vi "RT Driver VI.vi"(7 "Operation":T1, 11 "Device Reference in":T2 format="%.0x") -> (0 "Error Code":i32)   [LabVIEW 2016, in "FPGA Addon Engine.lvlib"]
uses:
  FPGA Addon Engine.lvlib
  <vilib>/NI Veristand/Custom Device API/Custom Device Item Ref.ctl
  <vilib>/NI Veristand/Custom Device API/Hardware Interface Driver VI Operation.ctl
  <vilib>/NI/NIVS Inline Async API/_VS Inline Async API/VS Inline Async API/VS Inline Async API.lvclass/VS Inline Async API.ctl
  <vilib>/NI/NIVS Inline Async API/_Data Access Engine/Data Access Engine/Data Access Engine.lvclass/Data Access Engine.ctl
  <vilib>/NI/NIVS Inline Async API/_Data Access Engine/Access Type Classes/Write/Write.lvclass/Write.ctl
  <vilib>/NI/NIVS Inline Async API/_Data Access Engine/Access Type Classes/ReadWrite/ReadWrite.lvclass/ReadWrite.ctl
  FPGA-Resource-Manager-APIs/Source/Shared/FPGA Settings.vi
  SubVIs/Initialize Scalar Datatypes and Refs.vi
  <vilib>/NI/NIVS Inline Async API/_Data Access Engine/Data Access Engine/Methods/Data.Engine.Read Data from HW.vi
  <vilib>/NI/NIVS Inline Async API/_VS Inline Async API/Error Handling Process/SubVIs/Error.GetError.vi
  <vilib>/NI/NIVS Inline Async API/_Data Access Engine/Access Type Classes/ReadWrite/ReadWrite.EngineData.vi
  <vilib>/NI/NIVS Inline Async API/_Data Access Engine/Access Type Classes/Write/Write.EngineData.vi
  <vilib>/NI Veristand/Custom Device API/NI VeriStand - Get Channel Value by Data Reference.vi
  <vilib>/NI Veristand/Custom Device API/NI VeriStand - Set Channel Value by Data Reference.vi
  <vilib>/Utility/config.llb/Open Config Data.vi
  <vilib>/Utility/config.llb/Get Key Names.vi
  <vilib>/Utility/config.llb/Write Key.vi
  <vilib>/Utility/config.llb/Write Key (I32).vi
  <vilib>/Utility/config.llb/Close Config Data.vi
  Shared/Constants.vi
  <vilib>/NI Veristand/Custom Device API/NI VeriStand - Get Item Property.vi
  <vilib>/NI Veristand/Custom Device API/Get Item Property (Variant).vi
  <vilib>/NI Veristand/Custom Device API/Get Item Property (Dependent File).vi
  <vilib>/NI Veristand/Custom Device API/Get Item Property (Path).vi
  <vilib>/NI Veristand/Custom Device API/Get Item Property (String).vi
  <vilib>/NI Veristand/Custom Device API/NI VeriStand - Set Item Property.vi
  <vilib>/NI Veristand/Custom Device API/Set Item Property (Path).vi
  <vilib>/NI Veristand/Custom Device API/Set Item Property (String).vi
  SubVIs/Initialize Input DMA Refs.vi
  SubVIs/Initialize Output DMA Refs.vi
  SubVIs/Initialize Scalar Datatype Classes.vi
  SubVIs/Output DMA Engine.vi
  <vilib>/Utility/error.llb/Error Cluster From Error Code.vi
  <vilib>/RVI Host/nirviSupport.llb/nirviErrorClusterFromErrorCode.vi
  <vilib>/rvi/errors/niLvFpgaAdjustHostInterfaceError.vi
  <vilib>/NI Veristand/Custom Device API/Global Data Refs.vi
  <vilib>/FPGAPlugInAG/Dynamic/niLvFpga_Close_Dynamic.vi
  <vilib>/NI Veristand/Custom Device Waveform API/Multiple Waveforms Write (DBL)/Multiple Waveforms Write (DBL).lvclass
  <vilib>/NI Veristand/Custom Device Waveform API/Single Waveform Read (DBL)/Single Waveform Read (DBL).lvclass
  <vilib>/NI/NIVS Inline Async API/_VS Inline Async API/VS Inline Async API/VS Inline Async API.lvclass
  <vilib>/rvi/interface/nirviMethod/nirviMethod.xnode
  <vilib>/rvi/interface/nirviCloseFPGA/nirviCloseFPGA.xnode
  <vilib>/NI VeriStand/Custom Device API/Custom Device API.lvlib
  <vilib>/NI VeriStand/Custom Device Tools/Custom Device Utility Library/Custom Device Utility Library.lvlib
  <vilib>/rvi/interface/nirviMethod/StockFPGA_InlinedMethodWaitForSingleIRQ.vi
  <vilib>/FPGAPlugInAG/Dynamic/niLvFpga_WaitOnIrq_Dynamic.vi
  <vilib>/FPGAPlugInAG/Dynamic/niLvFpga_AcknowledgeIrq_Dynamic.vi
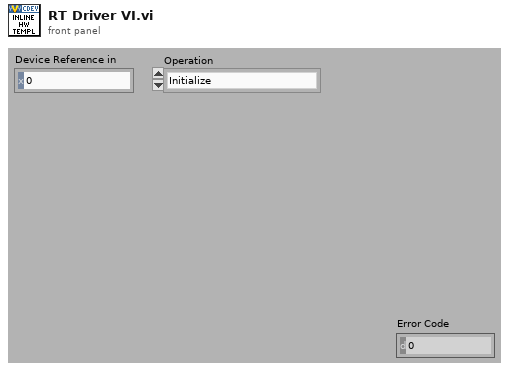
[diagram p1: front panel]
types:
  T1 = typedef "Custom Device API.lvlib/Hardware Interface Driver VI Operation.ctl" = enum16{"Initialize", "Start", "Read Data from HW", "Write Data to HW", "Close"}
  T2 = typedef "Custom Device API.lvlib/Custom Device Item Ref.ctl" = u64
  T3 = typedef "FPGA Addon Engine.lvlib/State Variables.ctl" = cluster{"FPGA Ref":refnum<k20>, "IncomingRegisters.Refs":T4[], "IncomingDMA.Refs":T7[], "OutgoingRegisters.Refs":T4[], "OutgoingDMA.Refs":T12[], "Compiled":T14}
  T4 = typedef "FPGA Addon Engine.lvlib/Register Settings.ctl" = cluster{"Data Type":T5, "U64":refnum<k20>, "U32":refnum<k20>, "U16":refnum<k20>, "U8":refnum<k20>, "I64":refnum<k20>, "I32":refnum<k20>, "I16":refnum<k20>, "I8":refnum<k20>, "SGL":refnum<k20>, "Bool":refnum<k20>, "Scalar Type":T6, "Index":i32, "Length":i32, "Analog PWM In":refnum<k20>, "Digital PWM In":refnum<k20>, "Digital PWM Out":refnum<k20>, "Analog PWM In Settings":refnum<k20>, "Digital PWM In Settings":refnum<k20>, "Sine Out":refnum<k20>, "FXP+/-24.5":refnum<k20>, "FXP+/-16.5":refnum<k20>, "FXP+/-32.8":refnum<k20>, "FXP+/-64.32":refnum<k20>, "FXP+/-16.7":refnum<k20>, "FXP+/-20.5":refnum<k20>}
  T5 = typedef "FPGA RM Shared API.lvlib/Data Type.ctl" = enum8{"<Null>", "I8", "I16", "I32", "I64", "U8", "U16", "U32", "U64", "SGL", "Boolean", "Analog PWM In Settings", "Analog PWM In", "Digital PWM In Settings", "Digital PWM In", "Digital PWM Out", "Sine Out", "FXP+/-24.5", "FXP+/-16.5", "FXP+/-32.8", "FXP+/-64.32", "FXP+/-16.7", "FXP+/-20.5"}
  T6 = typedef "FPGA Addon Shared.lvlib/Scalar Type.ctl" = enum16{"Standard", "Bitpacked"}
  T7 = typedef "FPGA Addon Engine.lvlib/DMA Input References.ctl" = cluster{"Waveform Ref":refnum<class "Multiple Waveforms Write (DBL).lvclass">, "DMA Ref":T8, "Name":string, "DMA Settings":T9}
  T8 = typedef "FPGA Addon Engine.lvlib/DMA Input Ref.ctl" = refnum<k20>
  T9 = typedef "FPGA Addon Shared.lvlib/DMA Settings.ctl" = cluster{"Number of Channels":u8, "Delacing Scheme":T10, "Update Rate":u32, "dt":dbl, "Mode":T11, "Number of Samples":u32, "DMA Host Buffer":u32}
  T10 = typedef "FPGA Addon Shared.lvlib/Delacing Scheme.ctl" = enum8{"Interleaved"}
  T11 = typedef "FPGA Addon Shared.lvlib/DMA Acquisition Mode.ctl" = enum8{"Continuous", "Triggered Finite"}
  T12 = typedef "FPGA Addon Engine.lvlib/DMA Output References.ctl" = cluster{"Waveforms":refnum<class "Single Waveform Read (DBL).lvclass">[], "DMA Ref":T13, "Name":string}
  T13 = typedef "FPGA Addon Engine.lvlib/DMA Output Ref.ctl" = refnum<k20>
  T14 = typedef "FPGA Addon Shared.lvlib/Compiled.Settings.ctl" = cluster{"Name":string, "IncomingRegisters.Settings":T15[], "IncomingRegisters.Refs":cluster{"Refs":T17[], "Values":dbl[]}, "OutgoingRegisters.Settings":T15[], "OutgoingRegisters.Refs":cluster{"Refs":T17[], "Values":dbl[]}, "Incoming.Size":i32, "Outgoing.Size":i32, "IncomingDMA.Settings":T19[], "OutgoingDMA.Settings":T19[], "FPGA.Settings":T21, "Target.Type":T22}
  T15 = typedef "FPGA Addon Shared.lvlib/Compiled.RegisterSettings.ctl" = cluster{"Scalar Type":T6, "Index":i32, "Length":i32, "Register":T16}
  T16 = typedef "FPGA Addon Shared.lvlib/Register Information.ctl" = cluster{"Name":string, "Data Type":T5, "Default Value":variant}
  T17 = typedef "Custom Device API.lvlib/Block Data Reference.ctl" = cluster{"Data Reference":T18, "Offset":u64, "Length":u64}
  T18 = typedef "Custom Device API.lvlib/Data Reference.ctl" = i32
  T19 = typedef "FPGA Addon Shared.lvlib/Compiled.DMASettings.ctl" = cluster{"Name":string, "DMA.Settings":T9, "DMA.VSRefs":T20[]}
  T20 = typedef "Custom Device API.lvlib/Waveform Data Reference.ctl" = i32
  T21 = typedef "FPGA RM Shared API.lvlib/FPGA Settings.ctl" = cluster{"Bitfile path":path, "RIO Device Address":string}
  T22 = typedef "Custom Device API.lvlib/Custom Device Target Type.ctl" = enum16{"PharLap", "VxWorks", "Windows", "Linux_32_ARM", "Linux_x64"}
  T23 = cluster{"Vars":T3, "Async?":bool, "Async":refnum<class "VS Inline Async API.lvclass">, "error out":errorcluster}
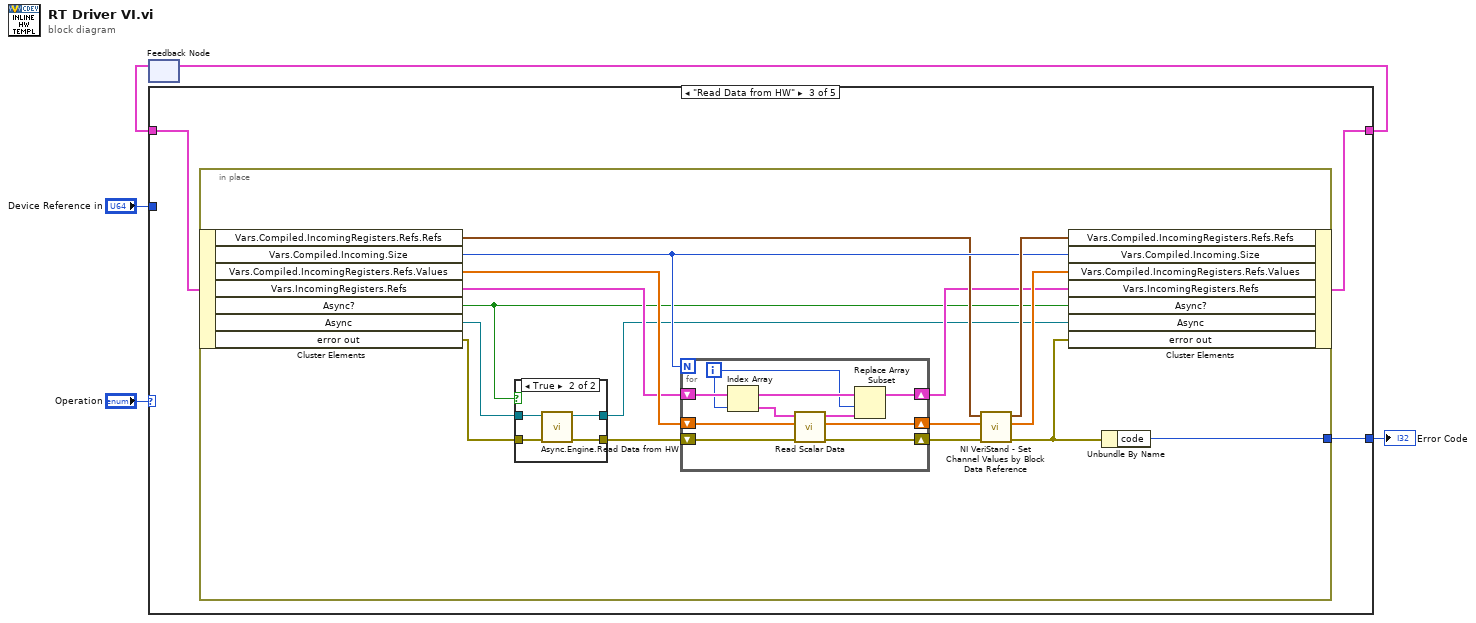
[diagram p0: block diagram]
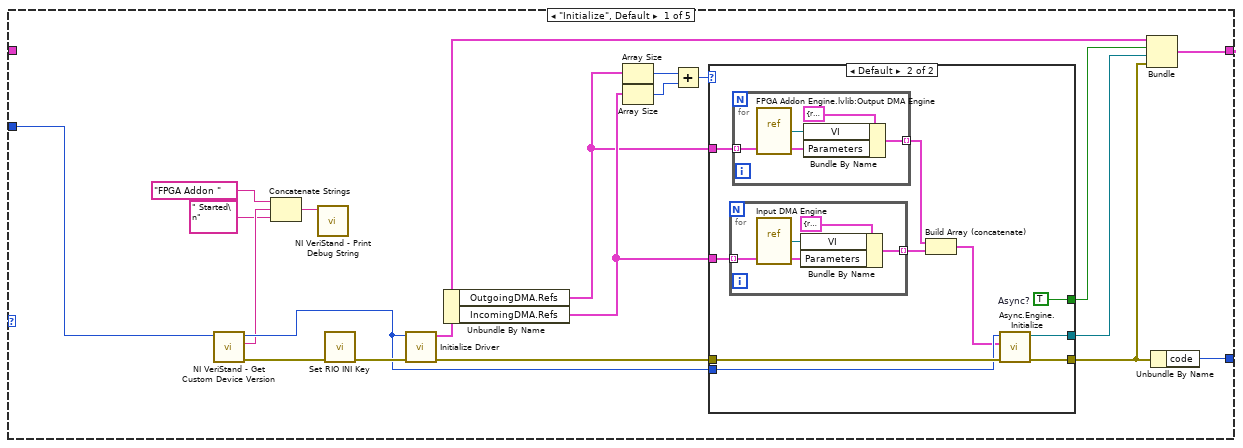
[diagram p2: hidden frame]
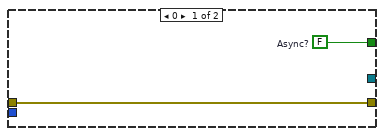
[diagram p3: hidden frame]
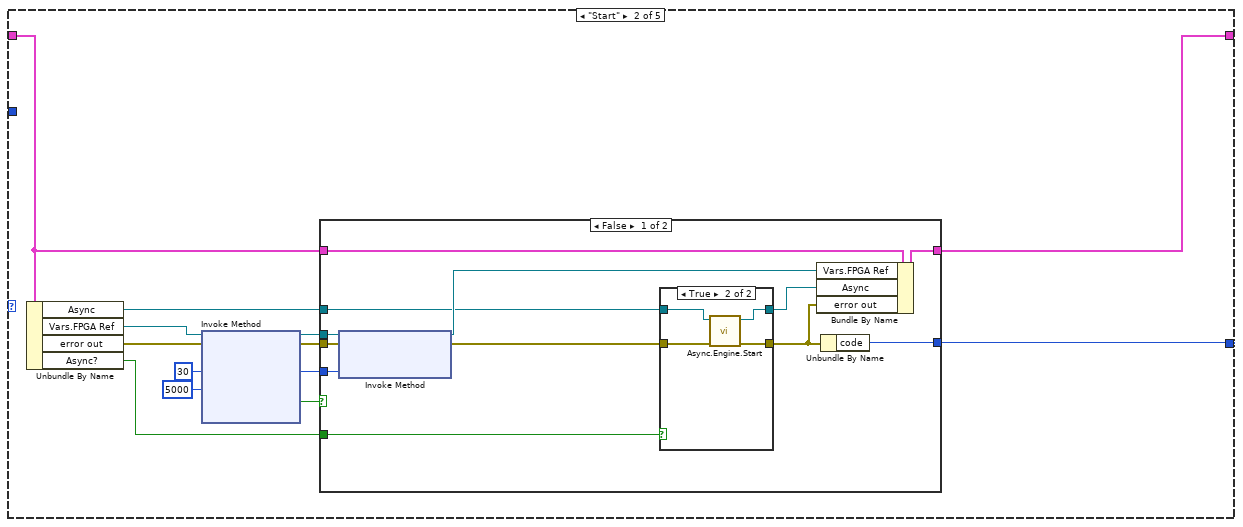
[diagram p4: hidden frame]
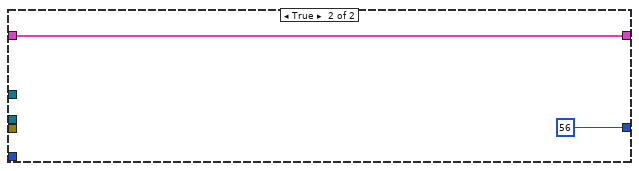
[diagram p6: hidden frame]
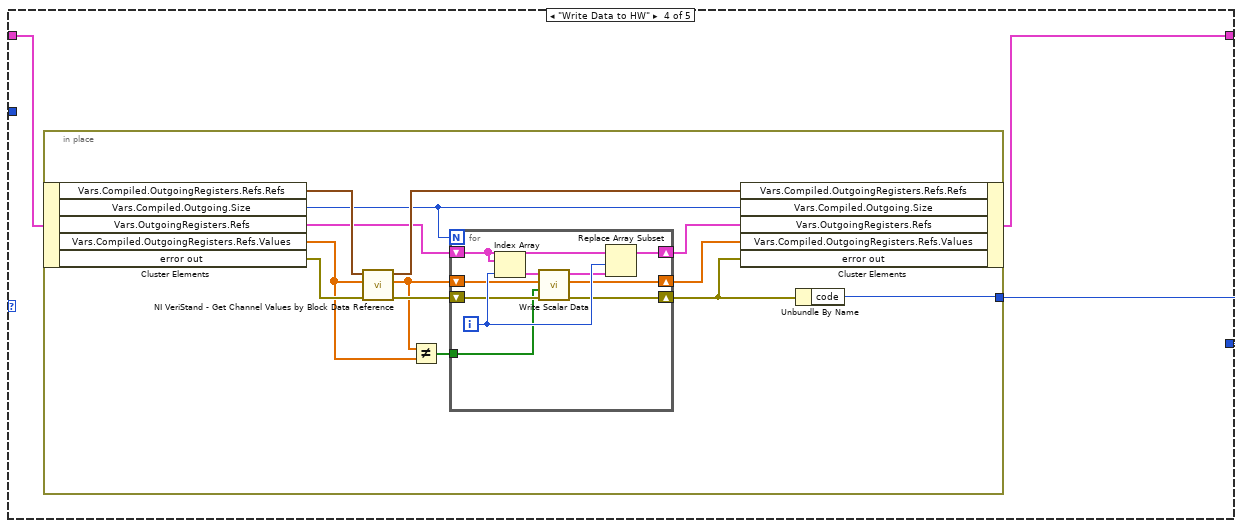
[diagram p8: hidden frame]
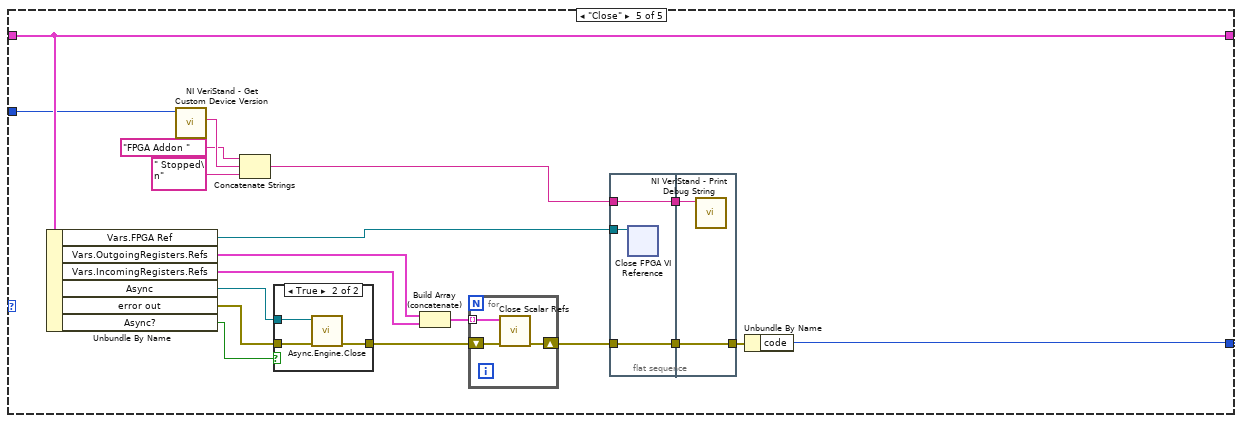
[diagram p9: hidden frame]
diagram:
  n1 = feedback #1() -> (w3:T23)  [unwired: 1 out]
  n2 = case shown="\"Read Data from HW\"" "Operation" {
    tunnel: [w25 w55 w80 w113 w154] -> w4
    tunnel: w3 -> [_ w56 w78 w114 w154]
    tunnel: "Device Reference in" -> [w11 _ _ _ w138]
    tunnel: [w24 w57 w79 w112 w156] -> w1
    frame "Initialize", Default {
      n3 = call <vilib>:"NI VeriStand - Get Custom Device Version.vi"("Device Ref in"=w11) -> ("error out"=w12:errorcluster, "Value"=w9:string, "Device Ref out"=w10:T2)  [unwired: 8 in]
      n4 = Concatenate Strings("FPGA Addon ", w9, " Started\n" ("string")) -> (w6:string)
      n5 = call <vilib>:"NI VeriStand - Print Debug String.vi"("Message"=w6) -> ()  [unwired: 10 in, 1 out]
      n6 = call "Set RIO INI Key.vi"("error in (no error)"=w12) -> ("error out"=w23:errorcluster)  [unwired: 10 in]
      n7 = call "Initialize Driver.vi"("error in (no error)"=w23, "Section Ref in"=w10) -> ("error out"=w22:errorcluster, "Vars"=w13:T3)  [unwired: 8 in]
      n8 = Unbundle By Name(w13) -> ("OutgoingDMA.Refs"=w18:T12[], "IncomingDMA.Refs"=w19:T7[])
      n9 = Array Size(array=w18) -> (size(s)=w17:i32)
      n10 = Array Size(array=w19) -> (size(s)=w16:i32)
      n11 = Add(x=w17, y=w16) -> (x+y=w15:i32)
      n12 = case shown="Default" w15 {
        tunnel: w22 -> [w27 w34]
        tunnel: [w27 w33] -> w21
        tunnel: [_ w32] -> w20
        tunnel: w19 -> [_ w30]
        tunnel: w18 -> [_ w37]
        tunnel: [w26 w35] -> w14
        tunnel: w10 -> [_ w31]
        frame 0 {
          w26 = FALSE  # Async?
        }
        frame Default {
          w35 = TRUE  # Async?
          n13 = for {
            tunnel: w30 -> [w40] mode=indexing
            tunnel: [w39] -> w29 mode=indexing
            n14 = vi-ref "Input DMA Engine.vi"() -> (w38:refnum<vi>)
            n15 = Bundle By Name(cluster=cluster{"VI":refnum<vi>, "Parameters":variant} {"VI"=refnum, "Parameters"=variant} ("Process"), "VI"=w38, "Parameters"=w40) -> (w39:cluster{"VI":refnum<vi>, "Parameters":variant})
          }
          n16 = for {
            tunnel: w37 -> [w44] mode=indexing
            tunnel: [w43] -> w36 mode=indexing
            n17 = vi-ref "FPGA Addon Engine.lvlib:Output DMA Engine.vi"() -> (w42:refnum<vi>)
            n18 = Bundle By Name(cluster=cluster{"VI":refnum<vi>, "Parameters":variant} {"VI"=refnum, "Parameters"=variant} ("Process"), "VI"=w42, "Parameters"=w44) -> (w43:cluster{"VI":refnum<vi>, "Parameters":variant})
          }
          n19 = Build Array (concatenate)(w36, w29) -> (w28:cluster{"VI":refnum<vi>, "Parameters":variant}[])
          n20 = call <vilib>:"Async.Engine.Initialize.vi"("error in (no error)"=w34, "Processes"=w28, "Custom Device Ref"=w31) -> ("error out"=w33:errorcluster, "Async"=w32:refnum<class "VS Inline Async API.lvclass">)  [unwired: 7 in]
        }
      }
      n21 = Bundle("Vars"=w13, "Async?"=w14, "Async"=w20, "error out"=w21) -> (w25:T23)  [unwired: 1 out]
      n22 = Unbundle By Name(w21) -> ("code"=w24:i32)
    }
    frame "Start" {
      w50 = 30 ("IRQ Number(s)")
      n23 = Unbundle By Name(w56) -> ("Async"=w46:refnum<class "VS Inline Async API.lvclass">, "Vars.FPGA Ref"=w54:refnum<k20>, "error out"=w53:errorcluster, "Async?"=w48:bool)
      n24 = xnode "Invoke Method"("FPGA VI Reference In"=w54, "error in"=w53, "IRQ Number(s)"=w50, "Timeout (ms)"=5000) -> ("FPGA VI Reference Out"=w52:refnum<k20>, "error out"=w51:errorcluster, "Timed Out"=w47:bool)  [unwired: 1 out]
      n25 = case shown="False" w47 {
        tunnel: [w69 56 ("code")] -> w57
        tunnel: w56 -> [w68 w77]
        tunnel: [w67 w77] -> w55
        tunnel: w52 -> [w66 _]
        tunnel: w51 -> [w65 _]
        tunnel: w50 -> [w64 _]
        tunnel: w48 -> [w61 _]
        tunnel: w46 -> [w60 _]
        frame False {
          n26 = xnode "Invoke Method"("FPGA VI Reference In"=w66, "error in"=w65, "IRQ Number(s)"=w64) -> ("FPGA VI Reference Out"=w63:refnum<k20>, "error out"=w58:errorcluster)
          n27 = case shown="True" w61 {
            tunnel: w58 -> [w71 w75]
            tunnel: [w71 w74] -> w62
            tunnel: w60 -> [w70 w73]
            tunnel: [w70 w72] -> w59
            frame False {
            }
            frame True {
              n28 = call <vilib>:"Async.Engine.Start.vi"("error in (no error)"=w75, "VS Inline Async API in"=w73) -> ("error out"=w74:errorcluster, "VS Inline Async API out"=w72:refnum<class "VS Inline Async API.lvclass">)  [unwired: 8 in]
            }
          }
          n29 = Bundle By Name(cluster=w68, "Vars.FPGA Ref"=w63, "Async"=w59, "error out"=w62) -> (w67:T23)
          n30 = Unbundle By Name(w62) -> ("code"=w69:i32)
        }
        frame True {
        }
      }
    }
    frame "Read Data from HW" {
      n31 = in-place {
        in-place-border: [w86] -> w79
        n32 = in-place-cluster #2(w78) -> ("Vars.Compiled.IncomingRegisters.Refs.Refs"=w90:T17[], "Vars.Compiled.Incoming.Size"=w92:i32, "Vars.Compiled.IncomingRegisters.Refs.Values"=w96:dbl[], "Vars.IncomingRegisters.Refs"=w89:T4[], "Async?"=w81:bool, "Async"=w83:refnum<class "VS Inline Async API.lvclass">, "error out"=w85:errorcluster)
        n33 = case shown="True" w81 {
          tunnel: w85 -> [w98 w102]
          tunnel: w83 -> [w97 w101]
          tunnel: [w98 w100] -> w84
          tunnel: [w97 w99] -> w82
          frame False {
          }
          frame True {
            n34 = call <vilib>:"Async.Engine.Read Data from HW.vi"("error in"=w102, "Async in"=w101) -> ("error out"=w100:errorcluster, "Async out"=w99:refnum<class "VS Inline Async API.lvclass">)  [unwired: 8 in]
          }
        }
        n35 = for {
          N: w92 -> [_]
          shift-right: [w103] -> w93
          shift-left: w96 -> [w104]
          shift-right: [w111] -> w88
          shift-left: w89 -> [w110]
          shift-right: [w108] -> w91
          shift-left: w84 -> [w109]
          i -> [w105]
          n36 = Index Array(array=w110, index=w105) -> (element=w106:T4)
          n37 = call "Read Scalar Data.vi"("error in (no error)"=w109, "Values"=w104, "Cluster"=w106) -> ("error out"=w108:errorcluster, "Values"=w103:dbl[], "Cluster"=w107:T4)  [unwired: 6 in]
          n38 = Replace Array Subset(array=w110, new element=w107, index=w105) -> (w111:T4[])
        }
        n39 = call <vilib>:"NI VeriStand - Set Channel Values by Block Data Reference.vi"("error in (no error)"=w91, "Values Array in"=w93, "Block Data Ref"=w90) -> ("error out"=w87:errorcluster, "Values Array out"=w94:dbl[], "Block Data Ref dup"=w95:T17[])  [unwired: 6 in]
        n40 = in-place-cluster #2("Vars.Compiled.IncomingRegisters.Refs.Refs"=w95, "Vars.Compiled.Incoming.Size"=w92, "Vars.Compiled.IncomingRegisters.Refs.Values"=w94, "Vars.IncomingRegisters.Refs"=w88, "Async?"=w81, "Async"=w82, "error out"=w87) -> (w80:T23)
        n41 = Unbundle By Name(w87) -> ("code"=w86:i32)
      }
    }
    frame "Write Data to HW" {
      n42 = in-place {
        in-place-border: [w118] -> w112
        n43 = in-place-cluster #3(w114) -> ("Vars.Compiled.OutgoingRegisters.Refs.Refs"=w127:T17[], "Vars.Compiled.Outgoing.Size"=w121:i32, "Vars.OutgoingRegisters.Refs"=w125:T4[], "Vars.Compiled.OutgoingRegisters.Refs.Values"=w116:dbl[], "error out"=w120:errorcluster)
        n44 = call <vilib>:"NI VeriStand - Get Channel Values by Block Data Reference.vi"("error in (no error)"=w120, "Values Array in"=w116, "Block Data Ref"=w127) -> ("error out"=w122:errorcluster, "Values Array out"=w117:dbl[], "Block Data Ref dup"=w126:T17[])  [unwired: 6 in]
        n45 = Not Equal?(x=w117, y=w116) -> (x != y?=w115:bool[])
        n46 = for {
          N: w121 -> [_]
          shift-right: [w129] -> w123
          shift-left: w117 -> [w130]
          shift-right: [w137] -> w124
          shift-left: w125 -> [w136]
          shift-right: [w132] -> w119
          shift-left: w122 -> [w133]
          tunnel: w115 -> [w128]
          i -> [w135]
          n47 = Index Array(array=w136, index=w135) -> (element=w131:T4)
          n48 = call "Write Scalar Data.vi"("error in (no error)"=w133, "Changed?"=w128, "Values"=w130, "Cluster"=w131) -> ("error out"=w132:errorcluster, "Values"=w129:dbl[], "Cluster"=w134:T4)  [unwired: 5 in]
          n49 = Replace Array Subset(array=w136, new element=w134, index=w135) -> (w137:T4[])
        }
        n50 = in-place-cluster #3("Vars.Compiled.OutgoingRegisters.Refs.Refs"=w126, "Vars.Compiled.Outgoing.Size"=w121, "Vars.OutgoingRegisters.Refs"=w124, "Vars.Compiled.OutgoingRegisters.Refs.Values"=w123, "error out"=w119) -> (w113:T23)
        n51 = Unbundle By Name(w119) -> ("code"=w118:i32)
      }
    }
    frame "Close" {
      n52 = Unbundle By Name(w154) -> ("Vars.FPGA Ref"=w146:refnum<k20>, "Vars.OutgoingRegisters.Refs"=w153:T4[], "Vars.IncomingRegisters.Refs"=w152:T4[], "Async"=w143:refnum<class "VS Inline Async API.lvclass">, "error out"=w151:errorcluster, "Async?"=w145:bool)
      n53 = call <vilib>:"NI VeriStand - Get Custom Device Version.vi"("Device Ref in"=w138) -> ("Value"=w142:string)  [unwired: 8 in, 2 out]
      n54 = Concatenate Strings("FPGA Addon ", w142, " Stopped\n" ("string")) -> (w139:string)
      n55 = case shown="True" w145 {
        tunnel: w151 -> [w157 w160]
        tunnel: [w157 w159] -> w150
        tunnel: w143 -> [_ w158]
        frame False {
        }
        frame True {
          n56 = call <vilib>:"Async.Engine.Close.vi"("error in (no error)"=w160, "Async in"=w158) -> ("error out"=w159:errorcluster)  [unwired: 8 in, 1 out]
        }
      }
      n57 = Build Array (concatenate)(w153, w152) -> (w155:T4[])
      n58 = for {
        tunnel: w155 -> [w166] mode=indexing
        shift-right: [w167] -> w144
        shift-left: w150 -> [w168]
        n59 = call "Close Scalar Refs.vi"("error in (no error)"=w168, "Cluster"=w166) -> ("error out"=w167:errorcluster)  [unwired: 9 in]
      }
      n60 = flat-sequence {
        tunnel: w139 -> [w162]
        tunnel: w144 -> [w163]
        tunnel: [w163] -> w148
        tunnel: [w162] -> w147
        tunnel: w146 -> [w161]
        tunnel: [w165] -> w149
        tunnel: w148 -> [w165]
        tunnel: w147 -> [w164]
        frame #0 {
          n61 = xnode "Close FPGA VI Reference"("FPGA VI Reference In"=w161) -> ()  [unwired: 1 in, 1 out]
        }
        frame #1 {
          n62 = call <vilib>:"NI VeriStand - Print Debug String.vi"("Message"=w164) -> ()  [unwired: 10 in, 1 out]
        }
      }
      n63 = Unbundle By Name(w149) -> ("code"=w156:i32)
    }
  }
  "Error Code" <- w1
  n64 = feedback-in #1(w4) -> ()
